vi "Write Available Channels.vi"(7 "All Daq Channels":tag[](array[tag]), 8 "error in (no error)":errorcluster, 9 "Used DAQChannels":tag[](array[tag]), 10 "DAQ Channel Info":T1, 11 "Sequencer in":refnum<class "Sequencer.lvclass">) -> (0 "error out":errorcluster, 3 "Sequencer out":refnum<class "Sequencer.lvclass">)   [LabVIEW 2015, in "Sequencer.lvlib" / "Sequencer.lvclass"]
uses:
  Sequencer.lvclass
  Daq Channel Info.ctl
  SequencerInfo.lvclass
  SequencerConfig.lvclass
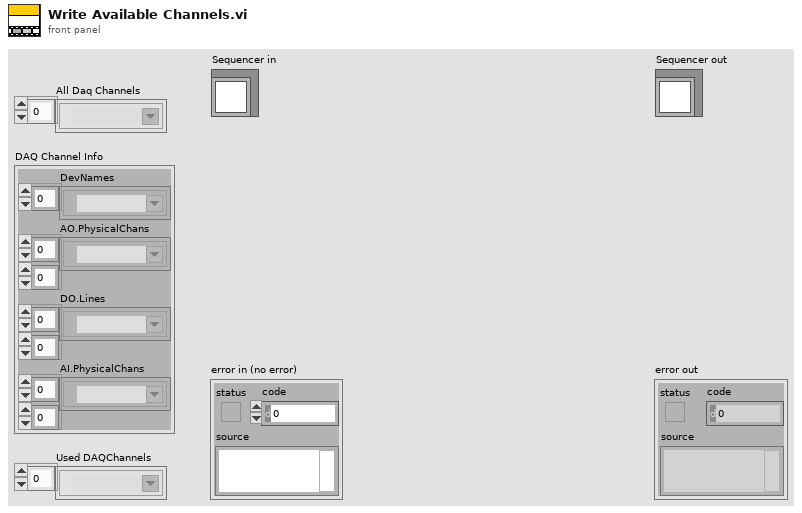
[diagram p1: front panel]
types:
  T1 = typedef "Sequencer.lvlib/Sequencer.lvclass/Daq Channel Info.ctl" = cluster{"DevNames":tag[], "AO.PhysicalChans":tag[][], "DO.Lines":tag[][], "AI.PhysicalChans":tag[][]}
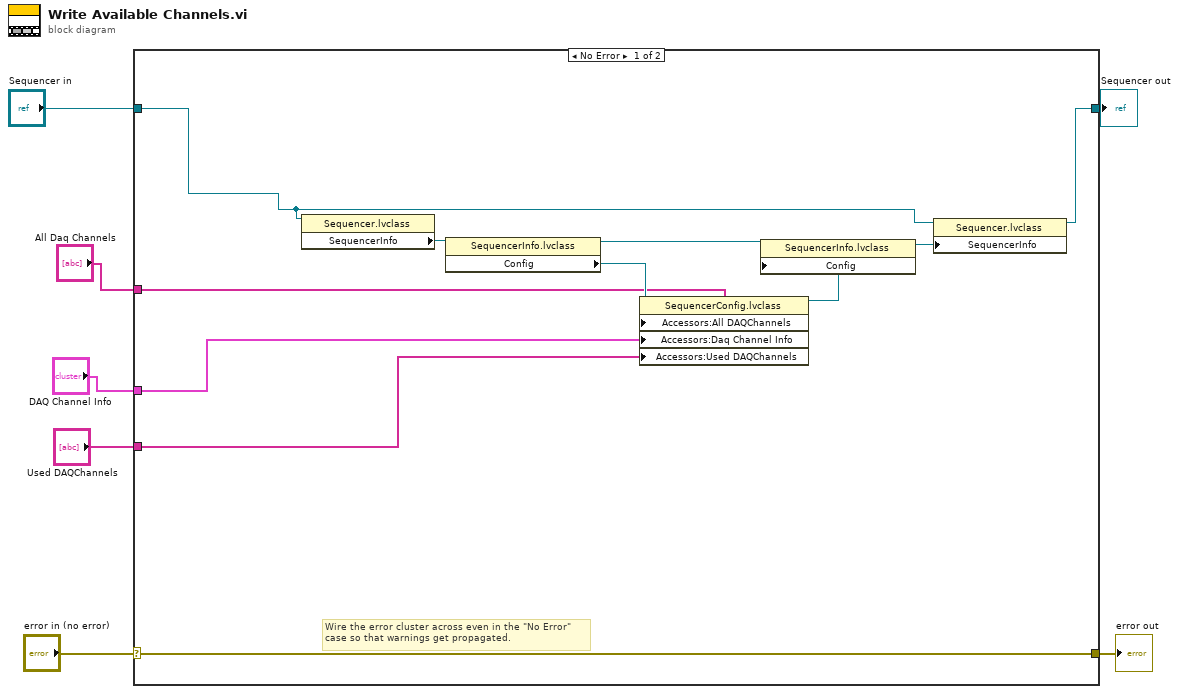
[diagram p0: block diagram]
diagram:
  n1 = case shown="No Error" "error in (no error)" {
    selector: "error in (no error)" -> [w18 w20]
    tunnel: [w18 w20] -> w6
    tunnel: [w11 w19] -> w4
    tunnel: "Sequencer in" -> [w12 w19]
    tunnel: "All Daq Channels" -> [w10 _]
    tunnel: "DAQ Channel Info" -> [w9 _]
    tunnel: "Used DAQChannels" -> [w8 _]
    frame No Error {
      # "Wire the error cluster across even in the \"No Error\"\ncase so that warnings get propagated."
      n2 = property class="Sequencer.lvclass"(reference=w12) -> ("SequencerInfo"=w13:refnum<class "SequencerInfo.lvclass">)  [unwired: 1 in, 2 out]
      n3 = property class="SequencerInfo.lvclass"(reference=w13) -> (reference out=w15:refnum<class "SequencerInfo.lvclass">, "Config"=w14:refnum<class "SequencerConfig.lvclass">)  [unwired: 1 in, 1 out]
      n4 = property class="SequencerConfig.lvclass"(reference=w14, "Accessors:All DAQChannels"=w10, "Accessors:Daq Channel Info"=w9, "Accessors:Used DAQChannels"=w8) -> (reference out=w16:refnum<class "SequencerConfig.lvclass">)  [unwired: 1 in, 1 out]
      n5 = property class="SequencerInfo.lvclass"(reference=w15, "Config"=w16) -> (reference out=w17:refnum<class "SequencerInfo.lvclass">)  [unwired: 1 in, 1 out]
      n6 = property class="Sequencer.lvclass"(reference=w12, "SequencerInfo"=w17) -> (reference out=w11:refnum<class "Sequencer.lvclass">)  [unwired: 1 in, 1 out]
    }
    frame Error {
    }
  }
  "error out" <- w6
  "Sequencer out" <- w4
